vi "thermometer.vi"(3 "lower_bound":dbl, 4 "upper_bound":dbl) -> (1 "Numeric":dbl)   [LabVIEW 2014]
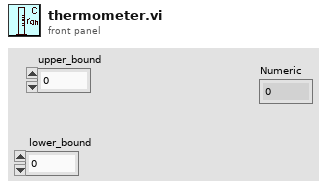
[diagram p1: front panel]
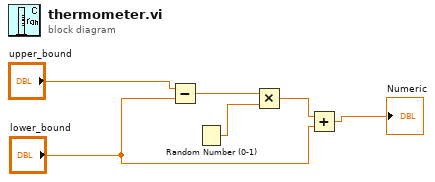
[diagram p0: block diagram]
diagram:
  n1 = Subtract(x="upper_bound", y="lower_bound") -> (x-y=w5:dbl)
  n2 = Random Number (0-1)() -> (number: 0 to 1=w4:dbl)
  n3 = Multiply(x=w5, y=w4) -> (x*y=w3:dbl)
  n4 = Add(x=w3, y="lower_bound") -> (x+y=→"Numeric":dbl)
